vi "MB_Relay_01_separated.vi"(10 "Array":bool[](array[boolean]), 11 "Mem_mapping in":u16[](array[numeric])) -> (2 "Mem Mapping out":u16[](array[numeric]))   [LabVIEW 2018, in "MB Relay.lvlib"]
uses:
  MB Relay.lvlib
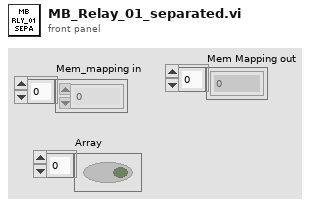
[diagram p1: front panel]
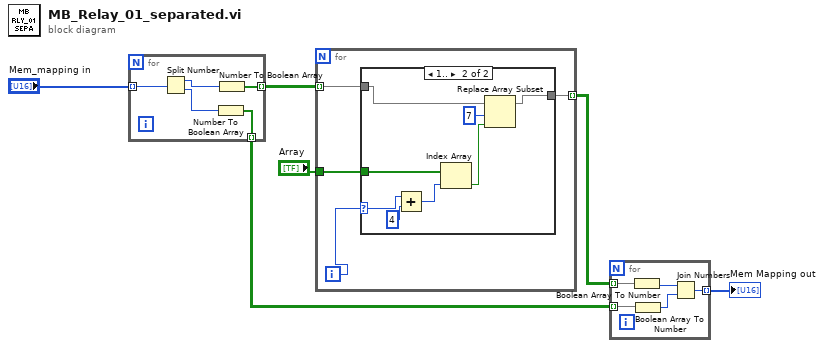
[diagram p0: block diagram]
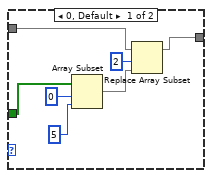
[diagram p2: hidden frame]
diagram:
  n1 = for {
    tunnel: "Mem_mapping in" -> [w10] mode=indexing
    tunnel: [w11] -> w4 mode=indexing
    tunnel: [w7] -> w2 mode=indexing
    n2 = Split Number(x=w10) -> (hi(x)=w9:u8, lo(x)=w8:u8)
    n3 = Number To Boolean Array(number=w8) -> (Boolean array=w7:bool[])
    n4 = Number To Boolean Array(number=w9) -> (Boolean array=w11:bool[])
  }
  n5 = for {
    tunnel: w4 -> [w14] mode=indexing
    tunnel: "Array" -> [w13]
    tunnel: [w12] -> w3 mode=indexing
    i -> [w15]
    n6 = case shown="1.." w15 {
      selector: w15 -> [_ w29]
      tunnel: w14 -> [w19 w26]
      tunnel: w13 -> [w22 w30]
      tunnel: [w16 w23] -> w12
      frame 0, Default {
        n7 = Array Subset(array=w22, index=0, length=5) -> (w18:bool[])
        n8 = Replace Array Subset(array=w19, new element=w18, index=2) -> (w16:bool[])
      }
      frame 1.. {
        n9 = Add(x=w29, y=4) -> (x+y=w27:i32)
        n10 = Index Array(array=w30, index=w27) -> (element=w24:bool)
        n11 = Replace Array Subset(array=w26, new element=w24, index=7) -> (w23:bool[])
      }
    }
  }
  n12 = for {
    tunnel: w3 -> [w35] mode=indexing
    tunnel: w2 -> [w34] mode=indexing
    tunnel: [w31] -> w1 mode=indexing
    n13 = Boolean Array To Number(Boolean array=w35) -> (number=w33:u8)
    n14 = Boolean Array To Number(Boolean array=w34) -> (number=w32:u8)
    n15 = Join Numbers(hi=w33, lo=w32) -> ((hi.lo)=w31:u16)
  }
  "Mem Mapping out" <- w1
